vi "Frequency Spectrum.vi"() -> ()   [LabVIEW 2013]
uses:
  <vilib>/Instr/_visa.llb/VISA Configure Serial Port (Instr).vi
panel:
  out "array":dbl[][](array[numeric])
  out "return code":i32
  out "standard error":string
  out "standard output":string
  out "Plot":T1(graph)
  out "error out 6":errorcluster
  in  "File Directory":path
  in  "Baud Rate":u32=9600
  in  "VISA resource name":refnum<visa-resource-name>
  in  "Start":bool
  out "error out 5":errorcluster
  out "error out 4":errorcluster
  in  "Increment Point":string
  out "read buffer":string
  out "error out 3":errorcluster
  in  "Ending Frequency":string
  out "error out 2":errorcluster
  in  "Staring Frequency":string
  out "error out":errorcluster
  in  "Stop":bool
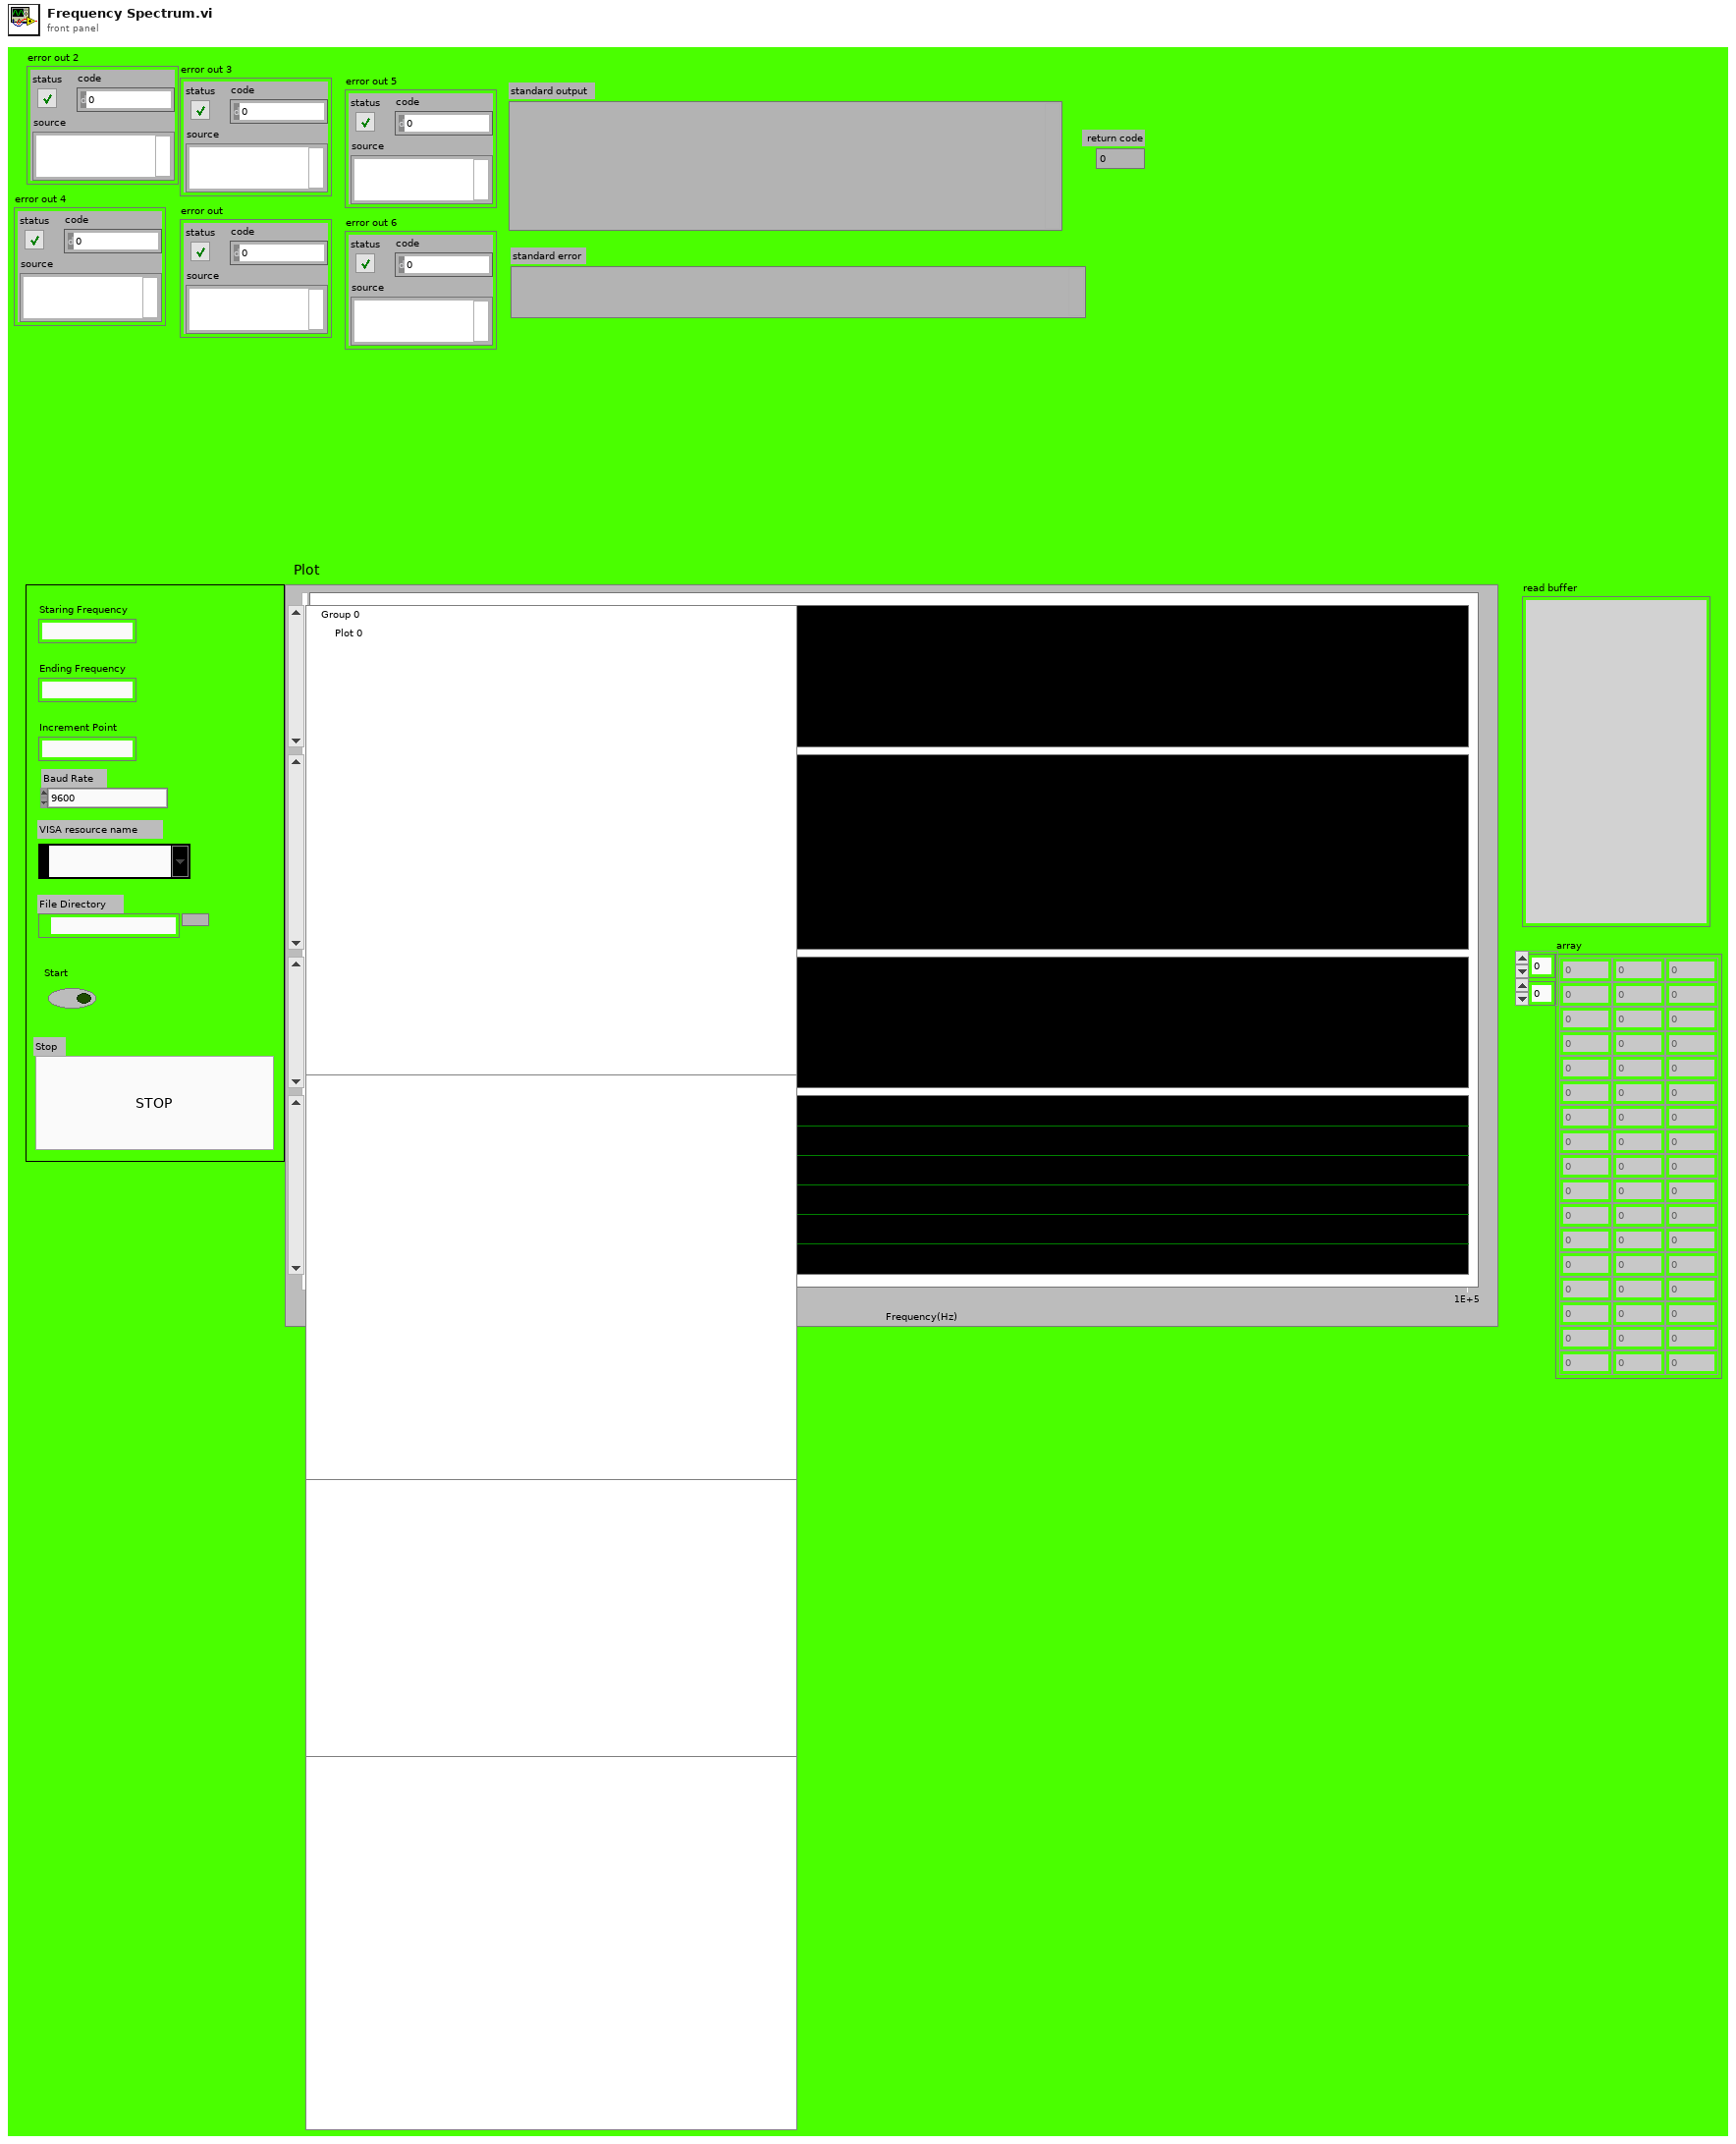
[diagram p1: front panel]
types:
  T1 = cluster{"array type (2D Dbl)":dbl[], "array type (2D Dbl)":dbl[]}[]
  T2 = cluster{"array type (2D Dbl)":dbl[], "array type (2D Dbl)":dbl[]}
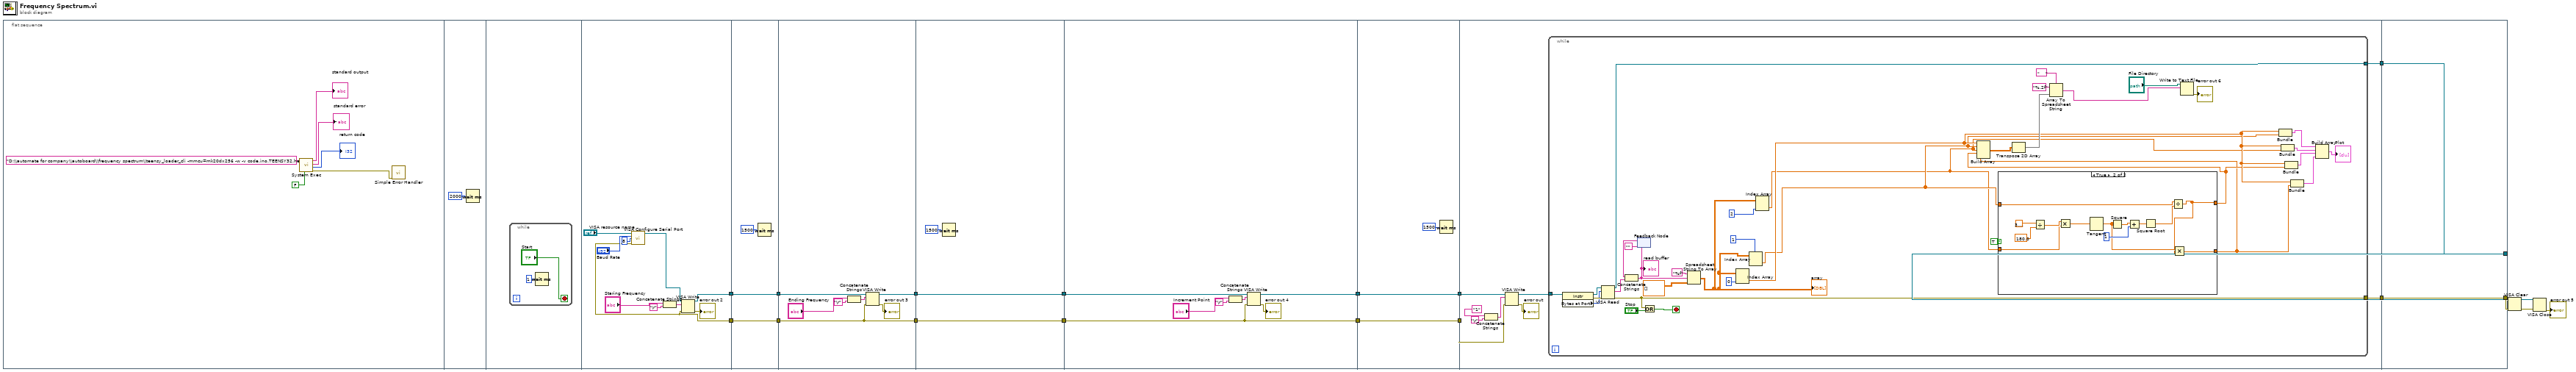
[diagram p0: block diagram]
diagram:
  n1 = flat-sequence {
    tunnel: [w37] -> w17
    tunnel: [w29] -> w15
    tunnel: w17 -> [w41]
    tunnel: [w41] -> w16
    tunnel: w15 -> [w40]
    tunnel: [w40] -> w14
    tunnel: w16 -> [w45]
    tunnel: [w47] -> w9
    tunnel: w14 -> [w46]
    tunnel: [w46] -> w7
    tunnel: w9 -> [w51]
    tunnel: [w51] -> w8
    tunnel: w7 -> [w50]
    tunnel: [w50] -> w6
    tunnel: w8 -> [w57]
    tunnel: [w56] -> w13
    tunnel: w6 -> [w55]
    tunnel: [w55] -> w11
    tunnel: w13 -> [w61]
    tunnel: [w61] -> w12
    tunnel: w11 -> [w60]
    tunnel: [w60] -> w10
    tunnel: w12 -> [w66]
    tunnel: [w70] -> w19
    tunnel: [w69] -> w18
    tunnel: w10 -> [w65]
    tunnel: [w122] -> w5
    tunnel: [w123] -> w4
    tunnel: w19 -> [w123]
    tunnel: w18 -> [w122]
    frame #0 {
      n2 = call <vilib>:"System Exec.vi"("run minimized? (F)"=FALSE, "command line"="D:\\automate for company\\autoboard\\frequency spectrum\\teensy_loader_cli -mmcu=mk20dx256 -w -v code.ino.TEENSY32.hex ") -> ("error out"=w21:errorcluster, "return code"=→"return code":i32, "standard error"=→"standard error":string, "standard output"=→"standard output":string)  [unwired: 6 in]
      n3 = call <vilib>:"Simple Error Handler.vi"("error in (no error)"=w21) -> ()  [unwired: 1 in, 8 out]
    }
    frame #1 {
      n4 = Wait (ms)(milliseconds to wait=u32 2000) -> ()  [unwired: 1 out]
    }
    frame #2 {
      n5 = while {
        stop <- "Start" stop-if-true
        n6 = Wait (ms)(milliseconds to wait=u32 1 ("대기 시간(ms)")) -> ()  [unwired: 1 out]
      }
    }
    frame #3 {
      n7 = call-poly "VISA Configure Serial Port"("VISA resource name"="VISA resource name", "baud rate (9600)"="Baud Rate", "data bits (8)"=u16 8) -> ("VISA resource name out"=w30:refnum<visa-resource-name>, "error out"=w29:errorcluster)  [unwired: 11 in]
      n8 = Concatenate Strings("Staring Frequency", "\r") -> (w35:string)
      n9 = VISA Write(VISA resource name=w30, write buffer=w35, error in (no error)=w29) -> (VISA resource name out=w37:refnum<visa-resource-name>, error out=→"error out 2":errorcluster)  [unwired: 1 out]
    }
    frame #4 {
      n10 = Wait (ms)(milliseconds to wait=u32 1500) -> ()  [unwired: 1 out]
    }
    frame #5 {
      n11 = Concatenate Strings("Ending Frequency", "\r") -> (w42:string)
      n12 = VISA Write(VISA resource name=w45, write buffer=w42, error in (no error)=w46) -> (VISA resource name out=w47:refnum<visa-resource-name>, error out=→"error out 3":errorcluster)  [unwired: 1 out]
    }
    frame #6 {
      n13 = Wait (ms)(milliseconds to wait=u32 1500) -> ()  [unwired: 1 out]
    }
    frame #7 {
      n14 = Concatenate Strings("Increment Point", "\r") -> (w52:string)
      n15 = VISA Write(VISA resource name=w57, write buffer=w52, error in (no error)=w55) -> (VISA resource name out=w56:refnum<visa-resource-name>, error out=→"error out 4":errorcluster)  [unwired: 1 out]
    }
    frame #8 {
      n16 = Wait (ms)(milliseconds to wait=u32 1500) -> ()  [unwired: 1 out]
    }
    frame #9 {
      n17 = Concatenate Strings("1" ("string"), "\r") -> (w63:string)
      n18 = VISA Write(VISA resource name=w66, write buffer=w63, error in (no error)=w65) -> (VISA resource name out=w67:refnum<visa-resource-name>, error out=→"error out":errorcluster)  [unwired: 1 out]
      n19 = while {
        tunnel: [w103] -> w70
        tunnel: [w100] -> w69
        tunnel: w67 -> [w99]
        stop <- w102 stop-if-true
        n20 = property on="Property Node" class="Instr"(reference=w99) -> (reference out=w105:refnum<visa-resource-name>, error out=w106:errorcluster, "Bytes at Port"=w104:u32)  [unwired: 1 in]
        n21 = VISA Read(VISA resource name=w105, byte count=w104, error in (no error)=w106) -> (VISA resource name out=w103:refnum<visa-resource-name>, read buffer=w96:string, error out=w100:errorcluster)  [unwired: 1 out]
        n22 = feedback #1("") -> (w97:string)
        n23 = Concatenate Strings(w97, w96) -> (w93:string)
        "read buffer" <- w93
        n24 = feedback-in #1(w93) -> ()
        n25 = Or(x=w100, y="Stop") -> (x .or. y?=w102:bool)
        n26 = Spreadsheet String To Array(format string="%f", spreadsheet string=w93, array type (2D Dbl)=dbl[][] []) -> (array=w89:dbl[][])  [unwired: 1 in]
        "array" <- w89
        n27 = Index Array(array=w89, index (col)=0 ("disabled index (col)")) -> (element=w75:dbl[])  [unwired: 1 in]
        n28 = Index Array(array=w89, index (col)=1 ("disabled index (col)")) -> (element=w72:dbl[])  [unwired: 1 in]
        n29 = Index Array(array=w89, index (col)=2 ("disabled index (col)")) -> (element=w71:dbl[])  [unwired: 1 in]
        n30 = case shown="True" TRUE {
          tunnel: w72 -> [w108 w112]
          tunnel: w71 -> [w107 w111]
          tunnel: [w107 w110] -> w73
          tunnel: [w108 w109] -> w74
          frame False {
          }
          frame True {
            n31 = Divide(x=3.141592653589793, y=180.0) -> (x/y=w119:dbl)
            n32 = Multiply(x=w119, y=w111) -> (x*y=w118:dbl[])
            n33 = Tangent(1:w118) -> (0:w113:dbl[])
            n34 = Square(x=w113) -> (x^2=w117:dbl[])
            n35 = Add(x=w117, y=1) -> (x+y=w115:dbl[])
            n36 = Square Root(x=w115) -> (sqrt(x)=w114:dbl[])
            n37 = Divide(x=w112, y=w114) -> (x/y=w109:dbl[])
            n38 = Multiply(x=w113, y=w109) -> (x*y=w110:dbl[])
          }
        }
        n39 = Build Array(w75, w72, w71, w74, w73) -> (w87:dbl[][])
        n40 = Transpose 2D Array(2D array=w87) -> (transposed array=w86:dbl[][])
        n41 = Array To Spreadsheet String(delimiter (Tab)="    ", array=w86, 3:"%.2f" ("format string")) -> (spreadsheet string=w82:string)
        n42 = Write to Text File(file (use dialog)="File Directory", text=w82) -> (error out=→"error out 6":errorcluster)  [unwired: 2 in, 2 out]
        n43 = Bundle("array type (2D Dbl)"=w75, "array type (2D Dbl)"=w72) -> (w80:T2)  [unwired: 1 in]
        n44 = Bundle("array type (2D Dbl)"=w75, "array type (2D Dbl)"=w71) -> (w79:T2)  [unwired: 1 in]
        n45 = Bundle("array type (2D Dbl)"=w75, "array type (2D Dbl)"=w74) -> (w78:T2)  [unwired: 1 in]
        n46 = Bundle("array type (2D Dbl)"=w75, "array type (2D Dbl)"=w73) -> (w77:T2)  [unwired: 1 in]
        n47 = Build Array(w80, w79, w78, w77) -> (→"Plot":T1)
      }
    }
    frame #10 {
    }
  }
  n48 = VISA Clear(VISA resource name=w4, error in (no error)=w5) -> (VISA resource name out=w2:refnum<visa-resource-name>, error out=w3:errorcluster)
  n49 = VISA Close(VISA resource name=w2, error in (no error)=w3) -> (error out=→"error out 5":errorcluster)
